vi "Generate Simulated Data.vi"(7 "Type de mode":bool, 8 "error in (no error)":T2 caption="entrée d'erreur (pas d'erreur)", 9 "Péri":tag="Dev1", 10 "Longueur d'onde":dbl, 11 "Type de signal":T1) -> (0 "error out":T2 caption="sortie d'erreur", 2 "Données du graphe":waveform(dbl)[](array[waveform]))   [LabVIEW 2018, in "Acquisition.lvlib"]
doc: "Génère des exemples de waveforms en fonction du type de signal dans l'entrée Configuration du matériel."
uses:
  Acquisition.lvlib
  Signal Type.ctl
  <vilib>/Analysis/NI_AALBase.lvlib
panel:
  out "Graphe déroulant":dynamicdata(graph)
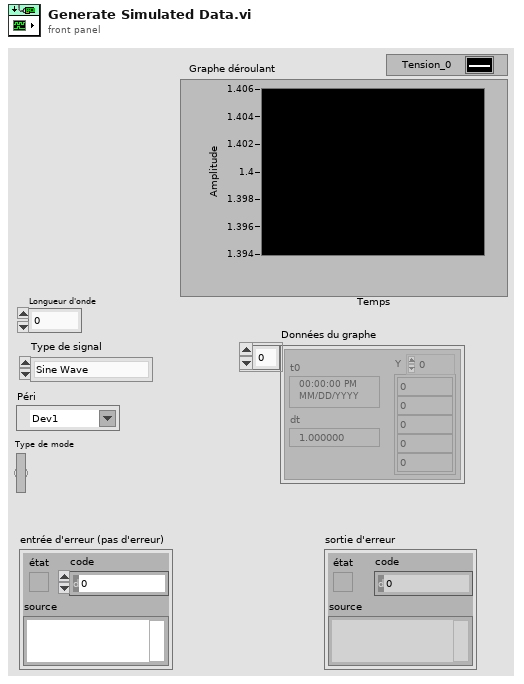
[diagram p1: front panel]
types:
  T1 = typedef "Acquisition.lvlib/Signal Type.ctl" = enum16{"Sine Wave", "Square with Noise", "Signal triangulaire", "Simulation DAQ"}
  T2 = cluster{"état":bool, "code":i32, "source":string}
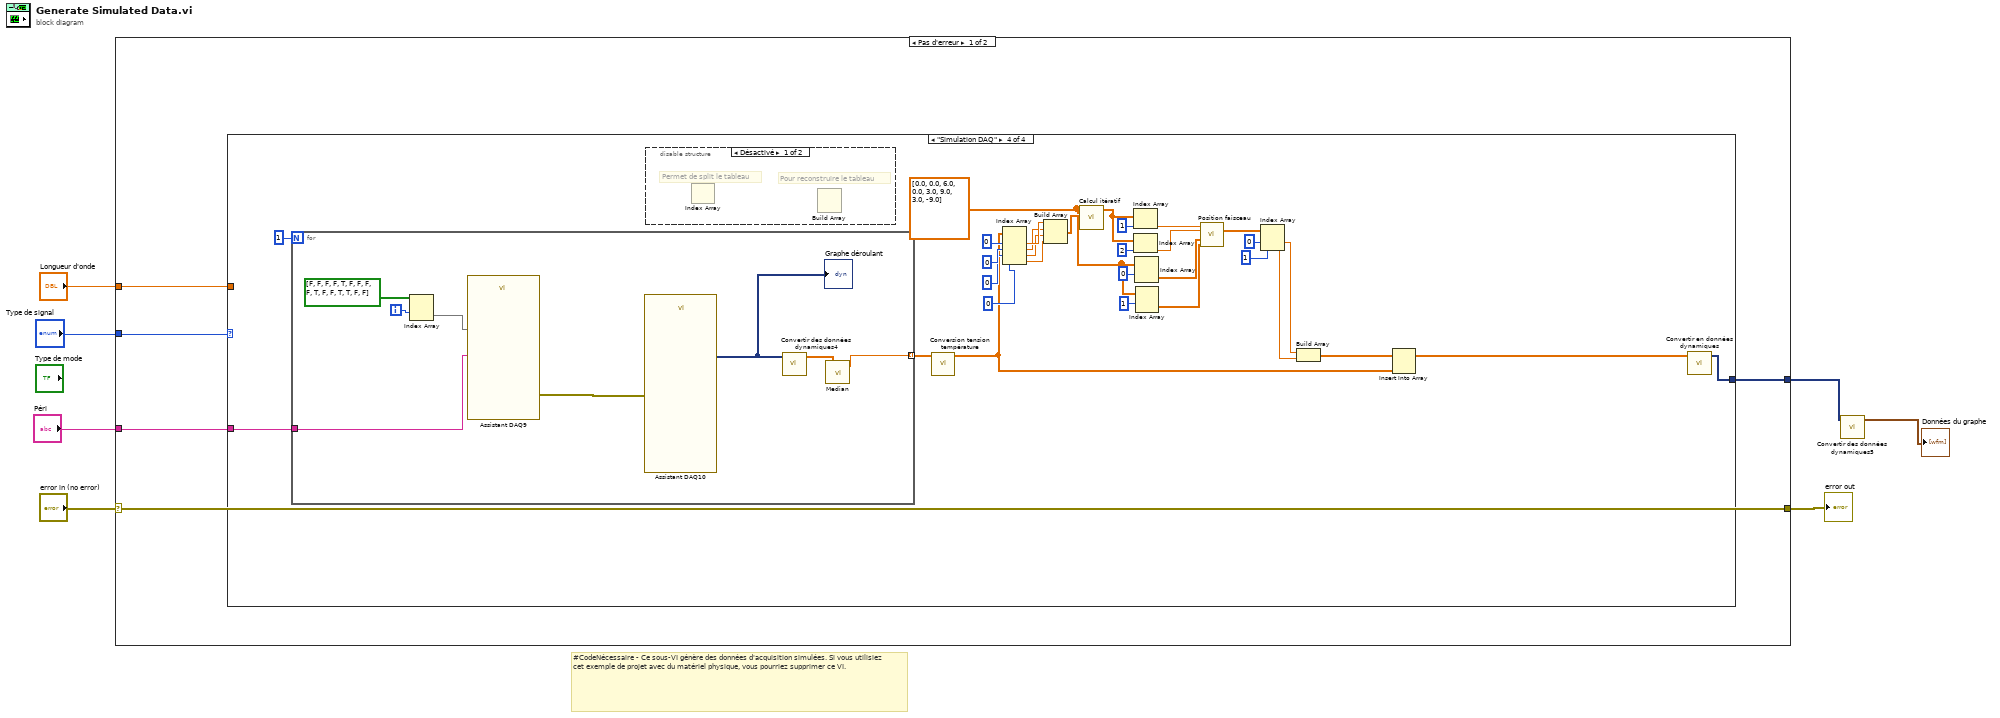
[diagram p0: block diagram]
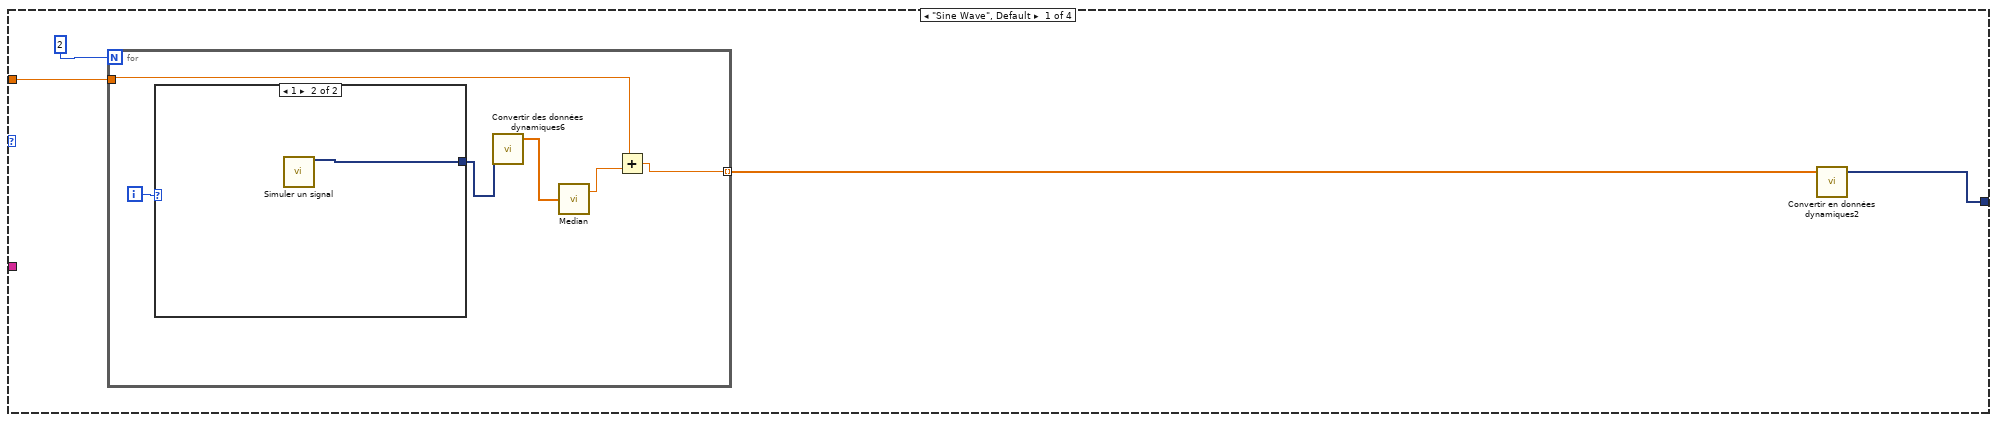
[diagram p2: hidden frame]
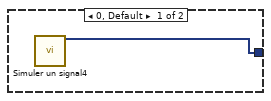
[diagram p3: hidden frame]
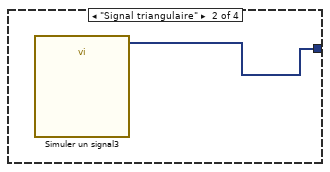
[diagram p4: hidden frame]
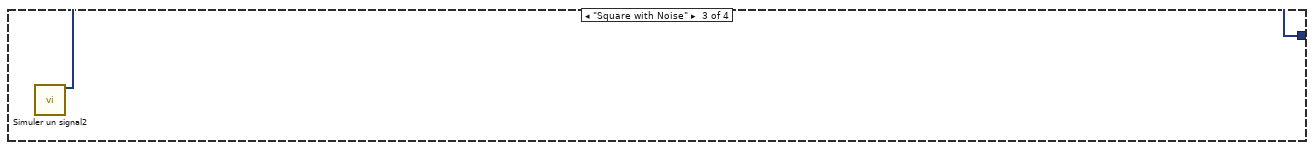
[diagram p5: hidden frame]
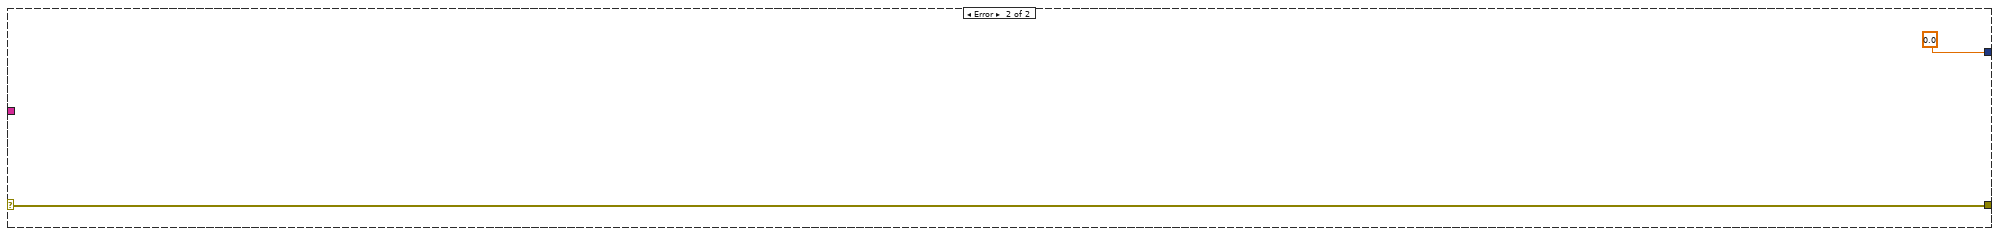
[diagram p7: hidden frame]
diagram:
  # "#CodeNécessaire - Ce sous-VI génère des données d'acquisition simulées. Si vous utilisiez cet exemple de projet avec du matériel physique, vous pourriez supprimer ce VI."
  n1 = case shown="Pas d'erreur" "error in (no error)" {
    selector: "error in (no error)" -> [w12 w67]
    tunnel: [w12 w67] -> w6
    tunnel: "Type de signal" -> [w11 _]
    tunnel: [w10 0.0] -> w3
    tunnel: "Longueur d'onde" -> [w9 _]
    tunnel: "Péri" -> [w8 _]
    frame No Error {
      n2 = case shown="\"Simulation DAQ\"" w11 {
        tunnel: [w15 w25 w26 w56] -> w10
        tunnel: w9 -> [w14 _ _ _]
        tunnel: w8 -> [_ _ _ w55]
        frame "Sine Wave", Default {
          n3 = for {
            N: 2 -> [_]
            tunnel: [w18] -> w13 mode=indexing
            tunnel: w14 -> [w17]
            i -> [w22]
            n4 = case shown="1" w22 {
              tunnel: [w23 w24] -> w21
              frame 0, Default {
                n5 = call "Simuler un signal4"() -> ("CC"=w23:dynamicdata)  [unwired: 14 in, 1 out]
              }
              frame 1 {
                n6 = call "Simuler un signal"() -> ("Sinus avec Bruit uniforme"=w24:dynamicdata)  [unwired: 14 in, 1 out]
              }
            }
            n7 = call "Convertir des données dynamiques6"("Dynamic Data Type"=w21) -> ("Array"=w20:dbl[])  [unwired: 3 in]
            n8 = call <vilib>:"Median.vi"("X"=w20) -> ("median"=w19:dbl)  [unwired: 1 out]
            n9 = Add(x=w17, y=w19) -> (x+y=w18:dbl)
          }
          n10 = call "Convertir en données dynamiques2"("Array"=w13) -> ("Dynamic Data Type"=w15:dynamicdata)  [unwired: 3 in]
        }
        frame "Signal triangulaire" {
          n11 = call "Simuler un signal3"() -> ("Triangle"=w25:dynamicdata)  [unwired: 14 in, 1 out]
        }
        frame "Square with Noise" {
          n12 = call "Simuler un signal2"() -> ("Square with Gaussian Noise"=w26:dynamicdata)  [unwired: 14 in, 1 out]
        }
        frame "Simulation DAQ" {
          w46 = dbl[][] [[0.0, 0.0], [6.0, 0.0], [3.0, 9.0], [3.0, -9.0]] ("Position des capteurs")
          n13 = for {
            N: 1 -> [_]
            tunnel: [w65] -> w41 mode=indexing
            tunnel: w55 -> [w58]
            i -> [w60]
            n14 = Index Array(array=bool[][] [[FALSE, FALSE, FALSE, FALSE], [TRUE, FALSE, FALSE, FALSE], [FALSE, TRUE, FALSE, FALSE], [TRUE, TRUE, FALSE, FALSE]], index (row)=w60) -> (element=w59:bool[])  [unwired: 1 in]
            n15 = call "Assistant DAQ9"("data"=w59, "nom du périphérique"=w58) -> ("error out"=w63:errorcluster)  [unwired: 16 in, 1 out]
            n16 = call "Assistant DAQ10"("error in"=w63) -> ("data"=w62:dynamicdata)  [unwired: 16 in, 2 out]
            "Graphe déroulant" <- w62
            n17 = call "Convertir des données dynamiques4"("Dynamic Data Type"=w62) -> ("Array"=w64:dbl[])  [unwired: 3 in]
            n18 = call <vilib>:"Median.vi"("X"=w64) -> ("median"=w65:dbl)  [unwired: 1 out]
          }
          n19 = disable-structure shown="Désactivé" {
            frame Disabled {
              # "Pour reconstruire le tableau"
              # "Permet de split le tableau"
              n20 = Index Array() -> ()  [unwired: 2 in, 1 out]
              n21 = Build Array() -> ()  [unwired: 4 in, 1 out]
            }
            frame Enabled {
            }
          }
          n22 = call "Conversion tension température.vi"("Data In"=w41) -> ("Data Out"=w27:dbl[])  [unwired: 10 in]
          n23 = Index Array(array=w27, index #1=0, index #2=0, index #3=0, index #4=0) -> (element #1=w53:dbl, element #2=w32:dbl, element #3=w31:dbl, element #4=w30:dbl)
          n24 = Build Array(w53, w32, w31, w30) -> (w54:dbl[])
          n25 = call "Calcul itératif.vi"("Température capteur 1-2-3-4-Ambiant"=w54, "Position des capteurs"=w46) -> ("DATA - T/R1/R2/R3"=w47:dbl[])  [unwired: 9 in]
          n26 = Index Array(array=w47, index=1 ("indice")) -> (element=w49:dbl)
          n27 = Index Array(array=w47, index=2 ("indice")) -> (element=w48:dbl)
          n28 = Index Array(array=w46, index (row)=0 ("indice (ligne)")) -> (element=w45:dbl[])  [unwired: 1 in]
          n29 = Index Array(array=w46, index (row)=1 ("indice (ligne)")) -> (element=w44:dbl[])  [unwired: 1 in]
          n30 = call "Position faisceau.vi"("R1"=w49, "R2"=w48, "Capteur 1"=w45, "Capteur 2"=w44) -> ("Coord"=w40:dbl[])  [unwired: 10 in, 1 out]
          n31 = Index Array(array=w40, index #1=0 ("indice"), index #2=1 ("indice")) -> (element #1=w37:dbl, element #2=w36:dbl)
          n32 = Build Array(w37, w36) -> (w28:dbl[])
          n33 = Insert Into Array(array=w28, new element=w27) -> (w29:dbl[])  [unwired: 1 in]
          n34 = call "Convertir en données dynamiques"("Array"=w29) -> ("Dynamic Data Type"=w56:dynamicdata)  [unwired: 3 in]
        }
      }
    }
    frame Error {
    }
  }
  "error out" <- w6
  n35 = call "Convertir des données dynamiques5"("Dynamic Data Type"=w3) -> ("Array of Waveform"=→"Données du graphe":waveform(dbl)[])  [unwired: 3 in]
